vi "Write.vi"(6 "Insert Timestamp Column (T)":bool=TRUE, 8 "error in (no error)":errorcluster, 10 "Message":string, 11 "Log in":refnum<class "Log.lvclass">) -> (0 "error out":errorcluster, 3 "Log out":refnum<class "Log.lvclass">)   [LabVIEW 2020, in "Log.lvclass"]
doc: "This VI writes a message the current file. After writing the message a check is done to see if the Max Lines has been reached, and starts a new file accordingly."
uses:
  Log.lvclass
  Log.lvclass/Log.ctl
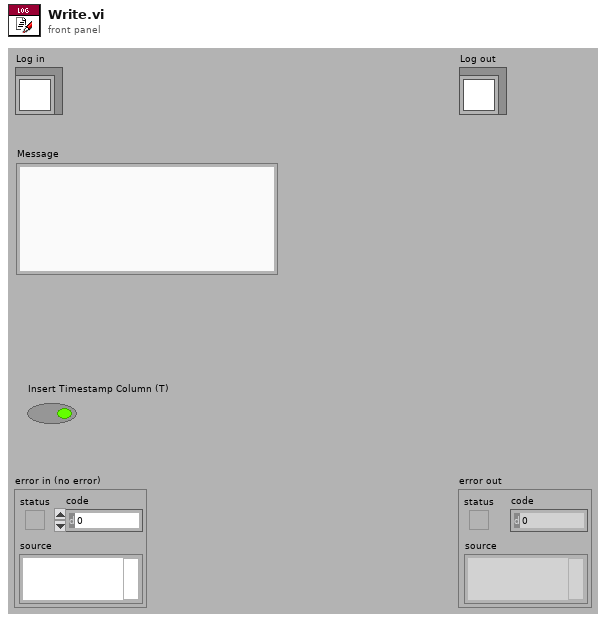
[diagram p1: front panel]
types:
  T1 = enum16{"open", "replace", "create", "open or create", "replace or create", "replace or create with confirmation"}
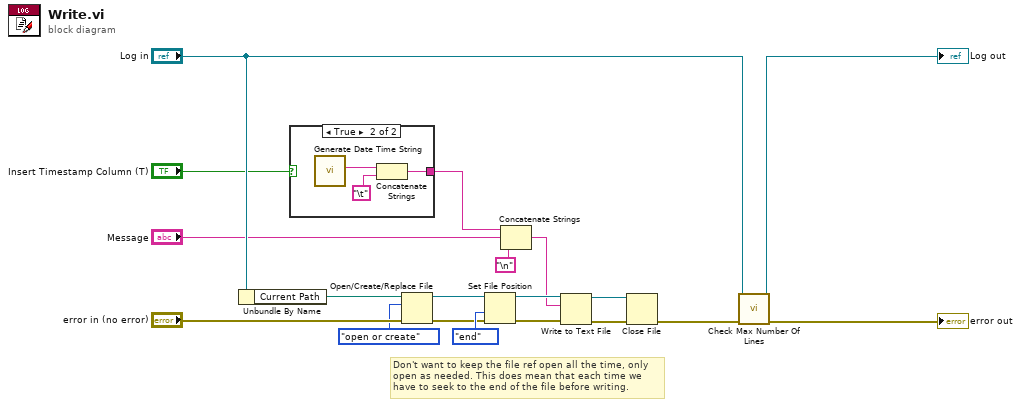
[diagram p0: block diagram]
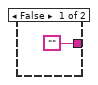
[diagram p2: hidden frame]
diagram:
  # "Don't want to keep the file ref open all the time, only open as needed. This does mean that each time we have to seek to the end of the file before writing."
  n1 = Unbundle By Name("Log in") -> ("Current Path"=w1:path)
  n2 = case shown="True" "Insert Timestamp Column (T)" {
    tunnel: ["" w22] -> w2
    frame False {
    }
    frame True {
      n3 = call "Generate Date Time String.vi"() -> ("Date time string with milliseconds"=w21:string)  [unwired: 10 in, 1 out]
      n4 = Concatenate Strings(w21, "\t") -> (w22:string)
    }
  }
  n5 = Open/Create/Replace File(file path (use dialog)=w1, error in="error in (no error)", operation (0:open)=T1."open or create") -> (refnum out=w13:refnum<file>, error out=w7:errorcluster)  [unwired: 4 out]
  n6 = Set File Position(refnum=w13, from (0:start)=enum16{"start", "end", "current"}."end", error in=w7) -> (refnum out=w11:refnum<file>, error out=w6:errorcluster)  [unwired: 1 out]
  n7 = Concatenate Strings(w2, "Message", "\n") -> (w9:string)
  n8 = Write to Text File(file (use dialog)=w11, text=w9, error in=w6) -> (refnum out=w8:refnum<file>, error out=w5:errorcluster)  [unwired: 2 out]
  n9 = Close File(refnum=w8, error in=w5) -> (error out=w3:errorcluster)  [unwired: 1 out]
  n10 = call "Check Max Number Of Lines.vi"("error in (no error)"=w3, "Log in"="Log in") -> ("error out"=→"error out":errorcluster, "Log out"=→"Log out":refnum<class "Log.lvclass">)  [unwired: 8 out]
